vi "Configure Channel.vi"(4 "Vertical Offset (0.0 V)":dbl format="%^.3e", 5 "Vertical Coupling (DC)":i32(slide)=1, 6 "Vertical Range (40 V)":dbl=40.0 format="%^.2e", 7 "Channel Enabled (True)":bool=TRUE, 8 "error in (no error)":errorcluster {"code" format="%.0x"}, 9 "Probe Attenuation (1x)":dbl=1.0 format="%.2f", 10 "Channel Name (\"Channel 1\")":string(combo)="CHAN1", 11 "VISA Resource Name":refnum<visa-resource-name>) -> (0 "error out":errorcluster {"code" format="%.0x"}, 3 "VISA Resource Name Out":refnum<visa-resource-name>)   [LabVIEW 2011, in "Agilent 546XX Series.lvlib"]
doc: "This VI configures the common properties of the oscilloscope's channel subsystem for a particular channel. These properties are the vertical range, vertical offset, coupling, probe attenuation, and channel enabled.\n\nNote: This VI has effect only on analog channels. If you want to configure digital channel, use VI ag546xx Configure Digital Channel instead."
uses:
  Agilent 546XX Series.lvlib
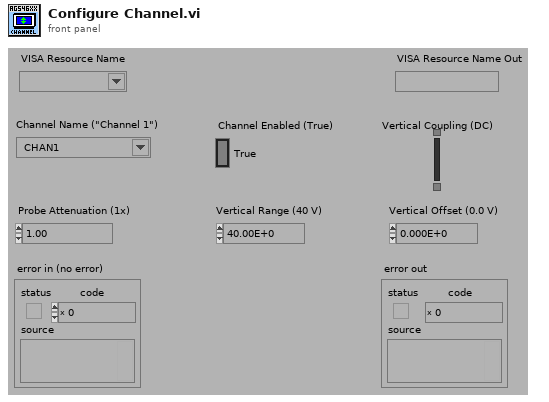
[diagram p1: front panel]
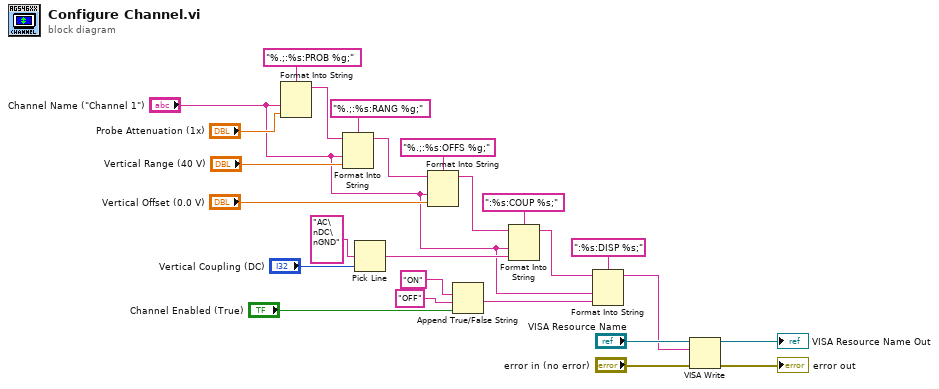
[diagram p0: block diagram]
diagram:
  n1 = Format Into String(format string="%.;:%s:PROB %g;", "Channel Name (\"Channel 1\")", "Probe Attenuation (1x)") -> (resulting string=w11:string)  [unwired: 2 in, 1 out]
  n2 = Format Into String(format string="%.;:%s:RANG %g;", initial string=w11, "Channel Name (\"Channel 1\")", "Vertical Range (40 V)") -> (resulting string=w18:string)  [unwired: 1 in, 1 out]
  n3 = Pick Line(multi-line string="AC\nDC\nGND", line index="Vertical Coupling (DC)") -> (output string=w6:string)  [unwired: 1 in]
  n4 = Format Into String(format string="%.;:%s:OFFS %g;", initial string=w18, "Channel Name (\"Channel 1\")", "Vertical Offset (0.0 V)") -> (resulting string=w15:string)  [unwired: 1 in, 1 out]
  n5 = Append True/False String(1:"Channel Enabled (True)", 2:"OFF" ("false string"), 3:"ON" ("true string")) -> (0:w2:string)  [unwired: 1 in]
  n6 = Format Into String(format string=":%s:COUP %s;", initial string=w15, "Channel Name (\"Channel 1\")", w6) -> (resulting string=w12:string)  [unwired: 1 in, 1 out]
  n7 = Format Into String(format string=":%s:DISP %s;", initial string=w12, "Channel Name (\"Channel 1\")", w2) -> (resulting string=w13:string)  [unwired: 1 in, 1 out]
  n8 = VISA Write(VISA resource name="VISA Resource Name", write buffer=w13, error in (no error)="error in (no error)") -> (VISA resource name out=→"VISA Resource Name Out":refnum<visa-resource-name>, error out=→"error out":errorcluster)  [unwired: 1 out]
